vi "Main Page.vi"(8 "error in (no error)":errorcluster, 11 "Node Ptr":T1 format="%.0x") -> (0 "error out":errorcluster)   [LabVIEW 2016, in "Untitled Project 1 System Explorer.lvlib"]
uses:
  Untitled Project 1 System Explorer.lvlib
  <vilib>/NI Veristand/Custom Device API/Custom Device Item Ref.ctl
  Shared/Constants.vi
  <vilib>/NI Veristand/Custom Device API/Get Item Property (String).vi
  <vilib>/NI Veristand/Custom Device API/Get Item Property (U16).vi
  <vilib>/NI Veristand/Custom Device API/Set Item Property (String).vi
  <vilib>/NI Veristand/Custom Device API/Set Item Property (U16).vi
  <vilib>/NI Veristand/Custom Device API/Custom Device API.lvlib
  Shared/Untitled Project 1 Shared.lvlib
panel:
  in  "Destination Port":u16
  in  "IP Address":string
  out "UDP Channels Transmitted":i32(listbox)
  in  "Header":cluster{"Section Name":string}={"Section Name"="Custom Device Item Settings"}
  in  "Description":string
  in  "Name":string
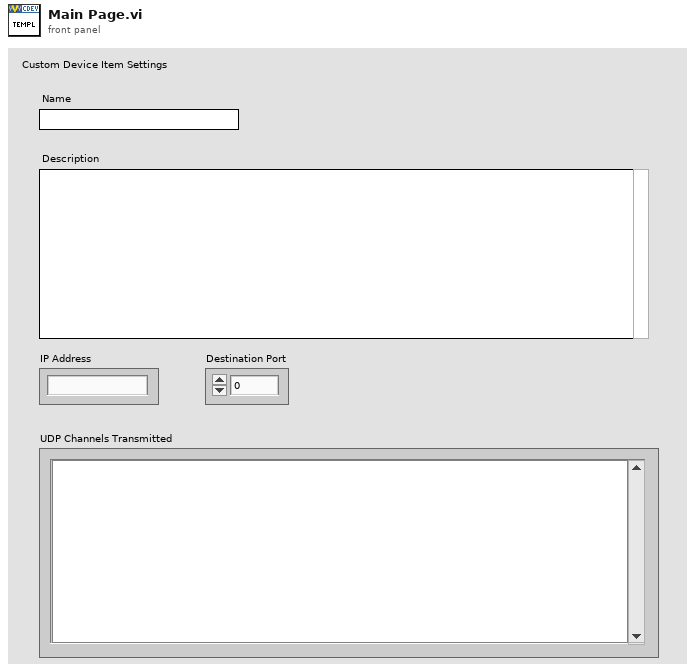
[diagram p1: front panel]
types:
  T1 = typedef "Custom Device API.lvlib/Custom Device Item Ref.ctl" = u64
  T2 = typedef "Custom Device API.lvlib/Custom Device Item Info.ctl" = cluster{"Name":string, "Is Channel":bool, "GUID":string, "Is Waveform":bool}
  T3 = typedef "Custom Device API.lvlib/Custom Device Commands.ctl" = enum16{"Default", "Item renamed", "Shutdown", "Dynamic button pressed"}
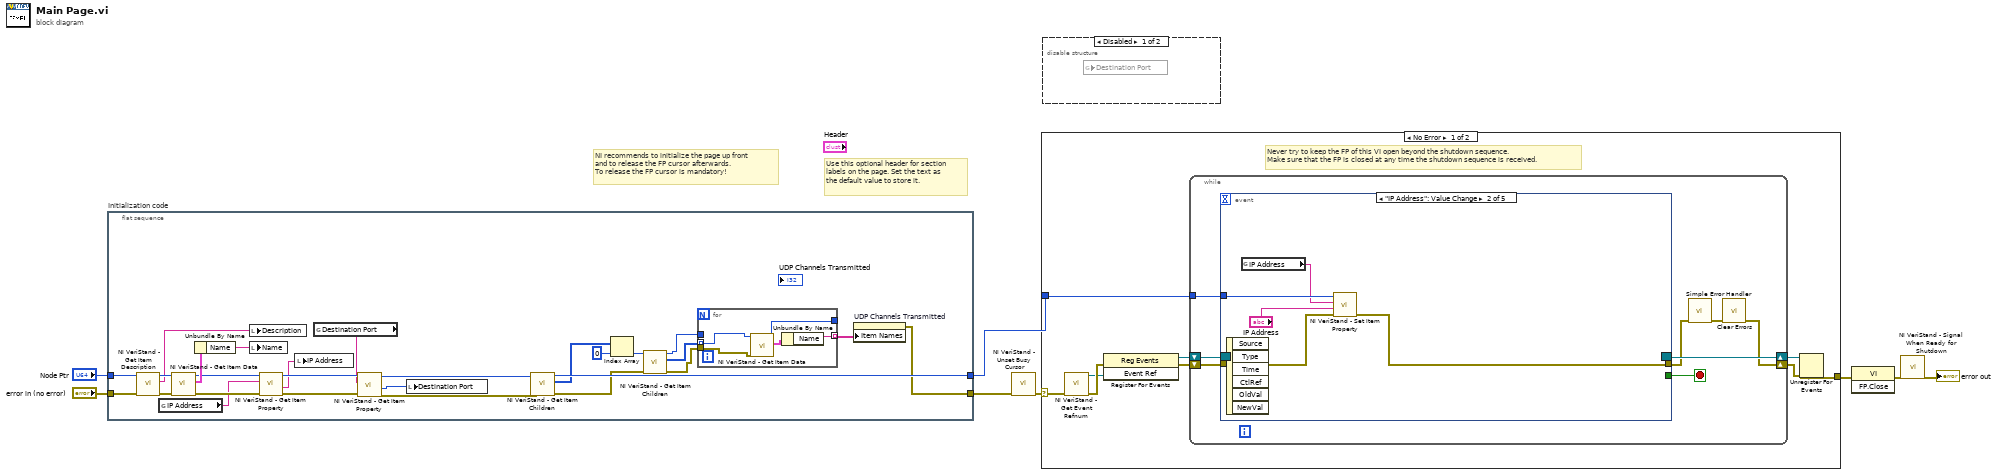
[diagram p0: block diagram]
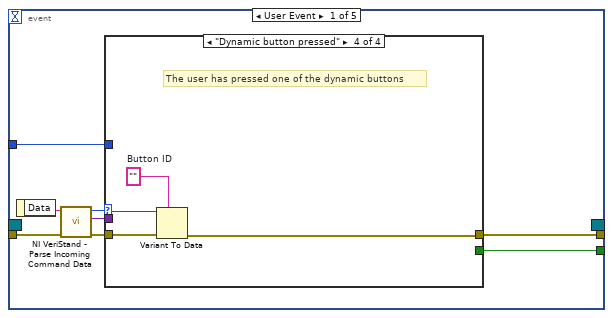
[diagram p3: hidden frame]
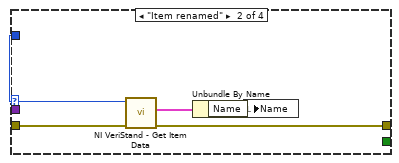
[diagram p5: hidden frame]
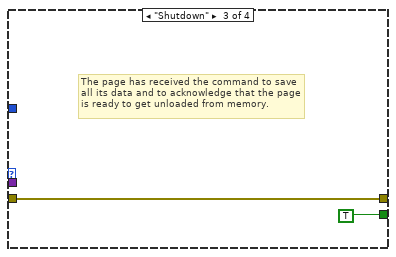
[diagram p6: hidden frame]
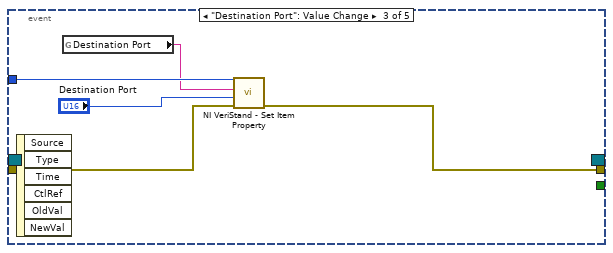
[diagram p7: hidden frame]
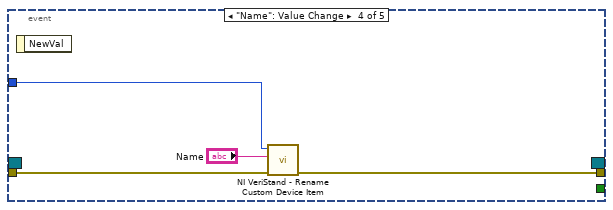
[diagram p8: hidden frame]
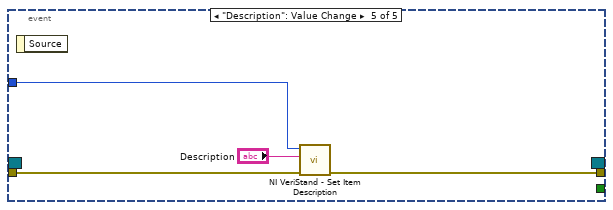
[diagram p9: hidden frame]
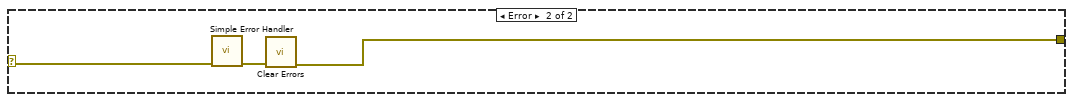
[diagram p10: hidden frame]
diagram:
  # "Use this optional header for section labels on the page. Set the text as the default value to store it."
  # "NI recommends to initialize the page up front\nand to release the FP cursor afterwards.\nTo release the FP cursor is mandatory!"
  n1 = flat-sequence "Initialization code" {
    tunnel: "error in (no error)" -> [w34]
    tunnel: "Node Ptr" -> [w33]
    tunnel: [w20] -> w4
    tunnel: [w28] -> w1
    frame #0 {
      n2 = call <vilib>:"NI VeriStand - Get Item Description.vi"("error in (no error)"=w34, "Item Ref in"=w33) -> ("error out"=w31:errorcluster, "Description"=w32:string, "Item Ref out"=w35:T1)  [unwired: 7 out]
      n3 = global read "Constants.vi" "IP Address"() -> (w16:string)
      n4 = call <vilib>:"NI VeriStand - Get Item Data.vi"("error in (no error)"=w31, "Item Ref in"=w35) -> ("error out"=w17:errorcluster, "Item Info"=w30:T2, "Item Ref out"=w18:T1)  [unwired: 7 out]
      n5 = Unbundle By Name(w30) -> ("Name"=w29:string)
      n6 = local write "Description"(w32) -> ()
      n7 = local write "Name"(w29) -> ()
      n8 = call-poly <vilib>:"NI VeriStand - Get Item Property.vi"("error in (no error)"=w17, "Property Name"=w16, "Item Ref in"=w18) -> ("error out"=w10:errorcluster, "Value"=w14:string, "Item Ref out"=w15:T1)  [unwired: 5 in, 1 out]
      n9 = local write "IP Address"(w14) -> ()
      n10 = global read "Constants.vi" "Destination Port"() -> (w13:string)
      n11 = call-poly <vilib>:"NI VeriStand - Get Item Property.vi"("error in (no error)"=w10, "Property Name"=w13, "Item Ref in"=w15) -> ("error out"=w9:errorcluster, "Value"=w11:u16, "Item Ref out"=w12:T1)  [unwired: 5 in, 1 out]
      n12 = local write "Destination Port"(w11) -> ()
      n13 = call <vilib>:"NI VeriStand - Get Item Children.vi"("error in (no error)"=w9, "Item Ref in"=w12) -> ("error out"=w24:errorcluster, "Child Refs"=w27:T1[], "Item Ref out"=w28:T1)  [unwired: 6 in, 1 out]
      n14 = Index Array(array=w27, index=0) -> (element=w25:T1)
      n15 = call <vilib>:"NI VeriStand - Get Item Children.vi"("error in (no error)"=w24, "Item Ref in"=w25) -> ("error out"=w21:errorcluster, "Child Refs"=w23:T1[], "Item Ref out"=w22:T1)  [unwired: 6 in, 1 out]
      n16 = for {
        tunnel: w23 -> [w40] mode=indexing
        tunnel: w22 -> [_]
        tunnel: w21 -> [w39]
        tunnel: [w38] -> _
        tunnel: [w36] -> w19 mode=indexing
        n17 = call <vilib>:"NI VeriStand - Get Item Data.vi"("error in (no error)"=w39, "Item Ref in"=w40) -> ("Item Info"=w37:T2, "Item Ref out"=w38:T1)  [unwired: 8 out]
        n18 = Unbundle By Name(w37) -> ("Name"=w36:string)
      }
      n19 = property on="UDP Channels Transmitted" class="LstBox (strict)"("Item Names"=w19) -> (error out=w20:errorcluster)  [unwired: 2 in, 1 out]
    }
  }
  n20 = call <vilib>:"NI VeriStand - Unset Busy Cursor.vi"("error in (no error)"=w4) -> ("error out"=w3:errorcluster)  [unwired: 10 out]
  n21 = case shown="No Error" w3 {
    selector: w3 -> [w41 w98]
    tunnel: [w46 w96] -> w8
    tunnel: w1 -> [w42 _]
    frame No Error {
      # "Never try to keep the FP of this VI open beyond the shutdown sequence.\nMake sure that the FP is closed at any time the shutdown sequence is received."
      n22 = call <vilib>:"NI VeriStand - Get Event Refnum.vi"("error in (no error)"=w41) -> ("error out"=w49:errorcluster, "Event Ref"=w45:refnum<user-event>)  [unwired: 9 out]
      n23 = register-events(error in=w49, w45) -> (reference out=w43:refnum<event-registration>, error out=w44:errorcluster)  [unwired: 1 in]
      n24 = while {
        tunnel: w42 -> [w53]
        shift-right: [w50] -> w47
        shift-left: w44 -> [w56]
        shift-right: [w57] -> w48
        shift-left: w43 -> [w55]
        stop <- w54 stop-if-true
        n25 = event shown="[1] \"IP Address\": Value Change" {
          selector: w55 -> [_ _ _ _ _]
          dyn-events: [_ _ _ _ _] -> w57
          timeout: _ -> [_ _ _ _ _]
          tunnel: w56 -> [w65 w80 w85 w91 w94]
          tunnel: [w61 _ _ _ _] -> w54
          tunnel: [w60 w79 w84 w90 w93] -> w52
          tunnel: w53 -> [w59 w82 w87 w89 w95]
          event User Event {
            n26 = event-data() -> ("Data"=w64:string)  [unwired: 1 out]
            n27 = call <vilib>:"NI VeriStand - Parse Incoming Command Data.vi"("error in (no error)"=w65, "Incoming data"=w64) -> ("error out"=w63:errorcluster, "Outgoing data"=w58:variant, "Action"=w62:T3)  [unwired: 7 out]
            n28 = case shown="\"Dynamic button pressed\"" w62 {
              tunnel: w63 -> [w66 w71 w72 w77]
              tunnel: [_ _ TRUE _] -> w61
              tunnel: [w66 w68 w72 w74] -> w60
              tunnel: w59 -> [_ w70 _ _]
              tunnel: w58 -> [_ _ _ w76]
              frame "Default", Default {
              }
              frame "Item renamed" {
                n29 = call <vilib>:"NI VeriStand - Get Item Data.vi"("error in (no error)"=w71, "Item Ref in"=w70) -> ("error out"=w68:errorcluster, "Item Info"=w69:T2)  [unwired: 8 out]
                n30 = Unbundle By Name(w69) -> ("Name"=w67:string)
                n31 = local write "Name"(w67) -> ()
              }
              frame "Shutdown" {
                # "The page has received the command to save all its data and to acknowledge that the page is ready to get unloaded from memory."
              }
              frame "Dynamic button pressed" {
                w75 = ""  # Button ID
                # "The user has pressed one of the dynamic buttons"
                n32 = Variant To Data(error in=w77, type=w75, Variant=w76) -> (error out=w74:errorcluster)  [unwired: 1 out]
              }
            }
          }
          event "IP Address": Value Change {
            n33 = event-data() -> ()  [unwired: 7 out]
            n34 = global read "Constants.vi" "IP Address"() -> (w81:string)
            n35 = call-poly <vilib>:"NI VeriStand - Set Item Property.vi"("error in (no error)"=w80, "Value"="IP Address", "Property Name"=w81, "Item Ref in"=w82) -> ("error out"=w79:errorcluster)  [unwired: 5 in, 2 out]
          }
          event "Destination Port": Value Change {
            n36 = event-data() -> ()  [unwired: 7 out]
            n37 = global read "Constants.vi" "Destination Port"() -> (w86:string)
            n38 = call-poly <vilib>:"NI VeriStand - Set Item Property.vi"("error in (no error)"=w85, "Value"="Destination Port", "Property Name"=w86, "Item Ref in"=w87) -> ("error out"=w84:errorcluster)  [unwired: 5 in, 2 out]
          }
          event "Name": Value Change {
            n39 = event-data() -> ()  [unwired: 2 out]
            n40 = call <vilib>:"NI VeriStand - Rename Custom Device Item.vi"("error in (no error)"=w91, "New Name"="Name", "Item Ref in"=w89) -> ("error out"=w90:errorcluster)  [unwired: 1 in, 7 out]
          }
          event "Description": Value Change {
            n41 = event-data() -> ()  [unwired: 2 out]
            n42 = call <vilib>:"NI VeriStand - Set Item Description.vi"("error in (no error)"=w94, "Description"="Description", "Item Ref in"=w95) -> ("error out"=w93:errorcluster)  [unwired: 8 out]
          }
        }
        n43 = call <vilib>:"Simple Error Handler.vi"("error in (no error)"=w52) -> ("error out"=w51:errorcluster)  [unwired: 1 in, 7 out]
        n44 = call <vilib>:"Clear Errors.vi"("error in (no error)"=w51) -> ("error out"=w50:errorcluster)  [unwired: 1 in, 5 out]
      }
      n45 = Unregister For Events(event registration refnum=w48, error in=w47) -> (error out=w46:errorcluster)
    }
    frame Error {
      n46 = call <vilib>:"Simple Error Handler.vi"("error in (no error)"=w98) -> ("error out"=w97:errorcluster)  [unwired: 1 in, 7 out]
      n47 = call <vilib>:"Clear Errors.vi"("error in (no error)"=w97) -> ("error out"=w96:errorcluster)  [unwired: 1 in, 5 out]
    }
  }
  n48 = disable-structure shown="Disabled" {
    frame Disabled {
      n49 = global read "Constants.vi" "Destination Port"() -> ()  [unwired: 1 in]
    }
    frame Enabled {
    }
  }
  n50 = invoke class="VI" method="FP.Close"(error in=w8) -> (error out=w7:errorcluster)  [unwired: 2 in, 2 out]
  n51 = call <vilib>:"NI VeriStand - Signal When Ready for Shutdown.vi"("error in (no error)"=w7) -> ("error out"=→"error out":errorcluster)  [unwired: 10 out]
